vi "v5.3.vi"() -> ()   [LabVIEW 2018]
uses:
  <vilib>/DAQmx/read.llb/DAQmx Read (Analog 1D DBL NChan 1Samp).vi
  <extravilib>/ChannelInstances/Lossy Stream-c(a[.](c(dbl,dbl,dbl,dbl)),stamp,a[.](dbl),c(dbl,dbl,dbl,dbl,dbl,dbl,dbl))/Read With Abort.vi
  <extravilib>/ChannelInstances/High Speed Stream-c(a[.](c(dbl,dbl,dbl,dbl)),stamp,a[.](dbl),c(dbl,dbl,dbl,dbl,dbl,dbl,dbl))/_Read For Replicate.vi
  <extravilib>/ChannelInstances/Lossy Stream-c(a[.](c(dbl,dbl,dbl,dbl)),stamp,a[.](dbl),c(dbl,dbl,dbl,dbl,dbl,dbl,dbl))/Write With Abort.vi
  <extravilib>/ChannelInstances/Lossy Stream-c(a[.](c(dbl,dbl,dbl,dbl)),stamp,a[.](dbl),c(dbl,dbl,dbl,dbl,dbl,dbl,dbl))/EndpointRead.vi
  <extravilib>/ChannelInstances/Lossy Stream-c(a[.](c(dbl,dbl,dbl,dbl)),stamp,a[.](dbl),c(dbl,dbl,dbl,dbl,dbl,dbl,dbl))/Endpoint.vi
  <extravilib>/ChannelInstances/Lossy Stream-c(a[.](c(dbl,dbl,dbl,dbl)),stamp,a[.](dbl),c(dbl,dbl,dbl,dbl,dbl,dbl,dbl))/Instantiate.vi
  <extravilib>/ChannelInstances/Lossy Stream-c(a[.](c(dbl,dbl,dbl,dbl)),stamp,a[.](dbl),c(dbl,dbl,dbl,dbl,dbl,dbl,dbl))/)Channel.vi
  <resource>/ChannelSupport/_ChannelSupport/WaitIfNeeded.vi
  <extravilib>/ChannelInstances/High Speed Stream-c(a[.](c(dbl,dbl,dbl,dbl)),stamp,a[.](dbl),c(dbl,dbl,dbl,dbl,dbl,dbl,dbl))/Instantiate.vi
  <extravilib>/ChannelInstances/High Speed Stream-c(a[.](c(dbl,dbl,dbl,dbl)),stamp,a[.](dbl),c(dbl,dbl,dbl,dbl,dbl,dbl,dbl))/)Channel.vi
  <extravilib>/ChannelInstances/High Speed Stream-c(a[.](c(dbl,dbl,dbl,dbl)),stamp,a[.](dbl),c(dbl,dbl,dbl,dbl,dbl,dbl,dbl))/Abort Signal/Init Signal.vi
  <vilib>/Utility/file.llb/Write Delimited Spreadsheet (string).vi
  <vilib>/DAQmx/create/channels.llb/DAQmx Create Channel (AI-Temperature-Thermocouple).vi
  <vilib>/DAQmx/configure/timing.llb/DAQmx Timing (Sample Clock).vi
  <vilib>/DAQmx/miscellaneous.llb/DAQmx Fill In Error Info.vi
  <extravilib>/ChannelInstances/High Speed Stream-c(a[.](c(dbl,dbl,dbl,dbl)),stamp,a[.](dbl),c(dbl,dbl,dbl,dbl,dbl,dbl,dbl)).lvlib
  <resource>/objmgr/daqmx.rc
  <extravilib>/ChannelInstances/Lossy Stream-c(a[.](c(dbl,dbl,dbl,dbl)),stamp,a[.](dbl),c(dbl,dbl,dbl,dbl,dbl,dbl,dbl)).lvlib
panel:
  out "DAQ Current Time":timestamp format="%<%X>T"
  in  "UI Refresh Rate (Hz)":u32=1 min=1 max=500 step=1
  out "Line Pressures":T1(graph)
  in  "Boondoggle":dbl(slide) scale=0.0..10.0
  out "Line Temperatures":T1(graph)
  out "Stoichiometric AFR [g/s]":dbl
  in  "stop":bool
  in  "Species List":string[][](table)=[["Custom", "9999999999"], ["Methanol", "6.47"], ["Butanol", "11.2"], ["Diesel", "14.5"], ["Gasoline", "14.7"], ["Propane", "15.67"], ["Methane", "13.19"], ["Hydrogen", "34.3"], ["Ammonia", "6.0466"], ["Pentane", "15.32"], ["Butane", "14.98"], ["Hexane", "15.24"], ["Ethanol", "9"], ["Empty (Not Used)", "0"]]
  in  "Lines Tab Control\n(Don't delete)":enum32{"Live Data", "AFR Info", "Setup Lines"}(tab)
  out "Flowrate Data":T2(array[cluster])
  out "AFR Display":T3(array[cluster])
  in  "Line Setup":T4(array[cluster])
  out "Actual Sample Rate":dbl
  out "Export Timestamp":timestamp format="%<%H:%M:%S>T"
  out "Rig Temperatures":T5
  out "UI Timestamp":timestamp format="%<%X\n%x>T"
  in  "file path (dialog if empty)":path
  out "Export Loop Status":T6(ring)
  in  "Start Recording?":bool
  in  "Stop Recording?":bool
  out "Aquisition\nLoop Status":T7(ring)
  in  "OK Button":bool
  in  "DAQ Properties":cluster{"Sample Rate [Hz]":dbl}={"Sample Rate [Hz]"=1.0} {"Sample Rate [Hz]" min=1.0 max=500.0 step=1.0}
  # "Live \n Live Line Data"
  # "Air-to-Fuel Ratios for each Line"
  # "Line Setup"
  # "Rig Temperatures [ °C]"
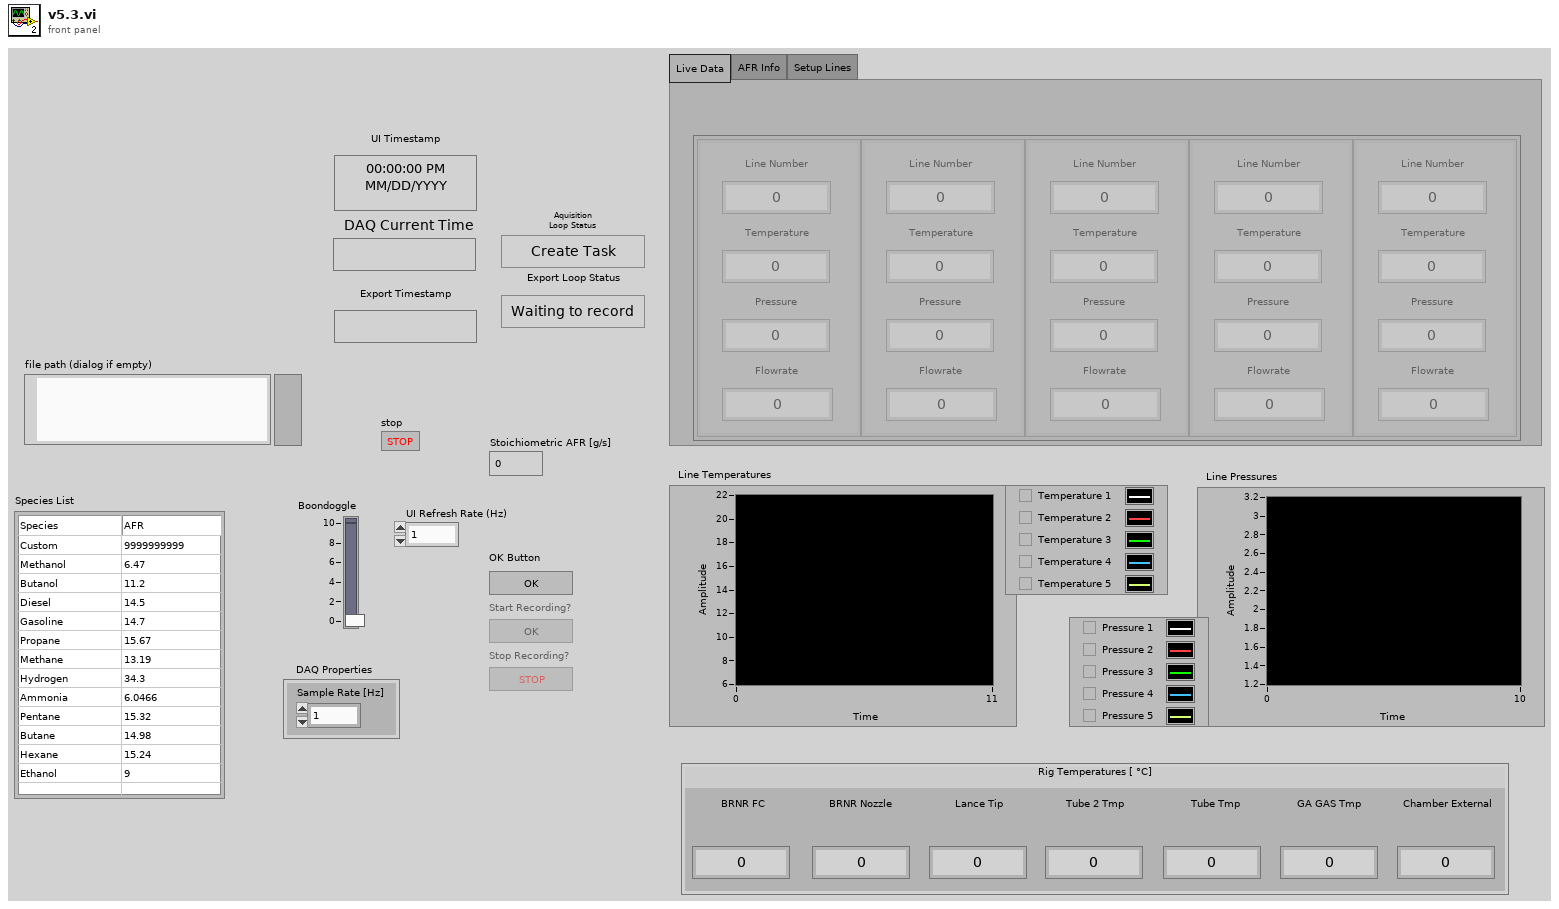
[diagram p1: front panel]
types:
  T1 = cluster{"[0]":dbl, "[1]":dbl, "[2]":dbl, "[3]":dbl, "[4]":dbl}
  T2 = cluster{"Line Number":dbl, "Temperature":dbl, "Pressure":dbl, "Flowrate":dbl}[]
  T3 = cluster{"Line Number":i32, "AFR":dbl, "Species":enum16{"Empty (Not used)", "Custom", "Methanol", "Ethanol", "Butanol", "Diesel", "Gasoline", "Propane", "Methane", "Hydrogen", "Pentane", "Butane", "Hexane"}}[]
  T4 = cluster{"Custom AFR":dbl, "Species":enum16{"Empty (Not used)", "Custom", "Methanol", "Ethanol", "Butanol", "Diesel", "Gasoline", "Propane", "Methane", "Hydrogen", "Pentane", "Butane", "Hexane"}}[]
  T5 = cluster{"BRNR FC":dbl, "BRNR Nozzle":dbl, "Lance Tip":dbl, "Tube 2 Tmp":dbl, "Tube Tmp":dbl, "GA GAS Tmp":dbl, "Chamber External":dbl}
  T6 = enum16{"Waiting to record", "Creating Spreadsheet", "Recording", "Finished Recording"}
  T7 = enum16{"Create Task", "Change Settings", "Check Settings", "Read Data", "End Task"}
  T8 = enum8{"Enabled", "Disabled", "Disabled and Grayed Out"}
  T9 = cluster{"Line":i32, "AFR":dbl, "Species":enum16{"Empty (Not used)", "Custom", "Methanol", "Ethanol", "Butanol", "Diesel", "Gasoline", "Propane", "Methane", "Hydrogen", "Pentane", "Butane", "Hexane"}}
  T10 = enum16{"Empty (Not used)", "Custom", "Methanol", "Ethanol", "Butanol", "Diesel", "Gasoline", "Propane", "Methane", "Hydrogen", "Pentane", "Butane", "Hexane"}
  T11 = cluster{"Flowrate Data":cluster{"Line Number":dbl, "Temperature":dbl, "Pressure":dbl, "Flowrate":dbl}[], "Current Time":timestamp, "DAQmx Data":dbl[], "Rig Temperatures":cluster{"BRNR FC":dbl, "BRNR Nozzle":dbl, "Lance Tip":dbl, "Tube 2 Tmp":dbl, "Tube Tmp":dbl, "GA GAS Tmp":dbl, "Chamber External Temp":dbl}}
  T12 = cluster{"BRNR FC":dbl, "BRNR Nozzle":dbl, "Lance Tip":dbl, "Tube 2 Tmp":dbl, "Tube Tmp":dbl, "GA GAS Tmp":dbl, "Chamber External Temp":dbl}
  T13 = typedef "High Speed Stream-c(a[.](c(dbl,dbl,dbl,dbl)),stamp,a[.](dbl),c(dbl,dbl,dbl,dbl,dbl,dbl,dbl)).lvlib/)Channel.ctl" = refnum<queue>
  T14 = typedef "Lossy Stream-c(a[.](c(dbl,dbl,dbl,dbl)),stamp,a[.](dbl),c(dbl,dbl,dbl,dbl,dbl,dbl,dbl)).lvlib/)Channel.ctl" = refnum<queue>
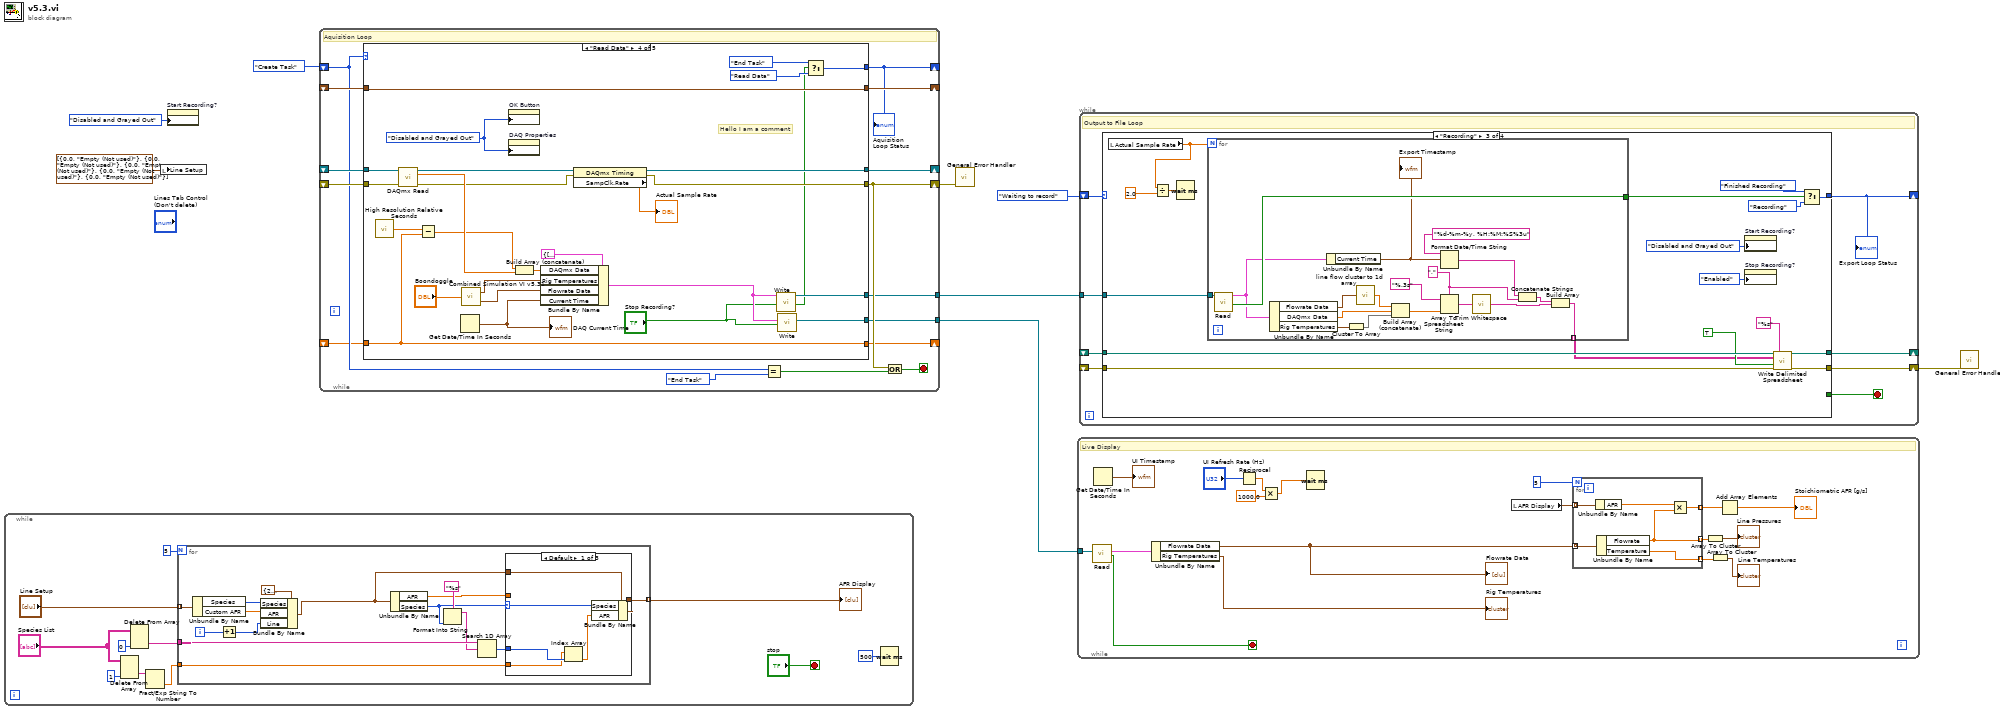
[diagram p0: block diagram]
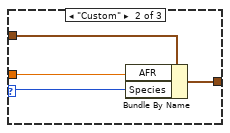
[diagram p2: hidden frame]
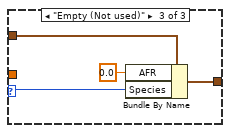
[diagram p3: hidden frame]
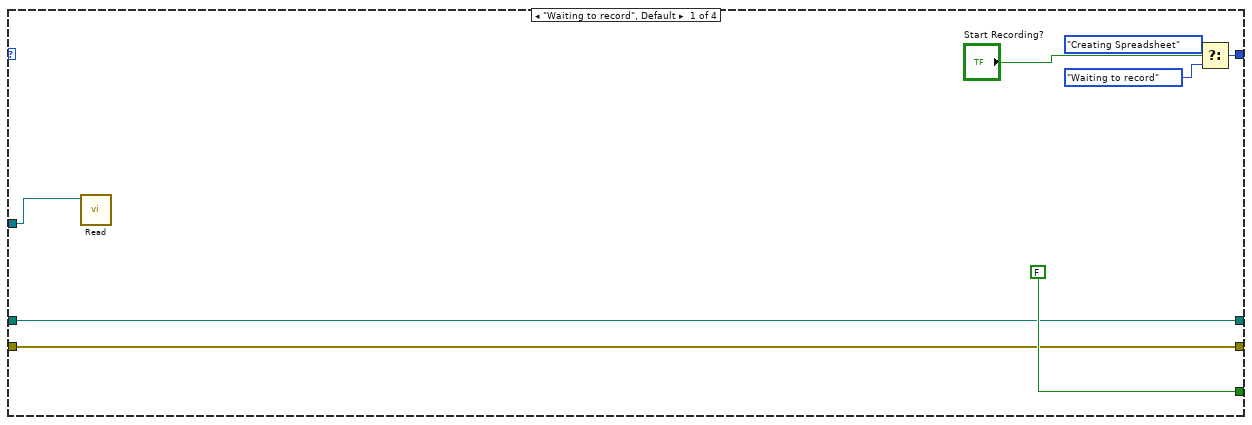
[diagram p4: hidden frame]
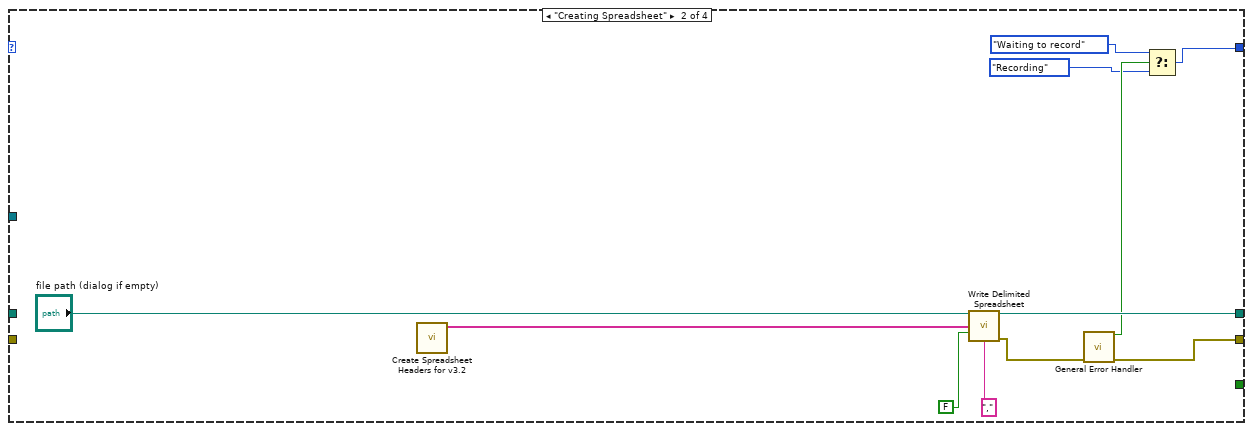
[diagram p5: hidden frame]
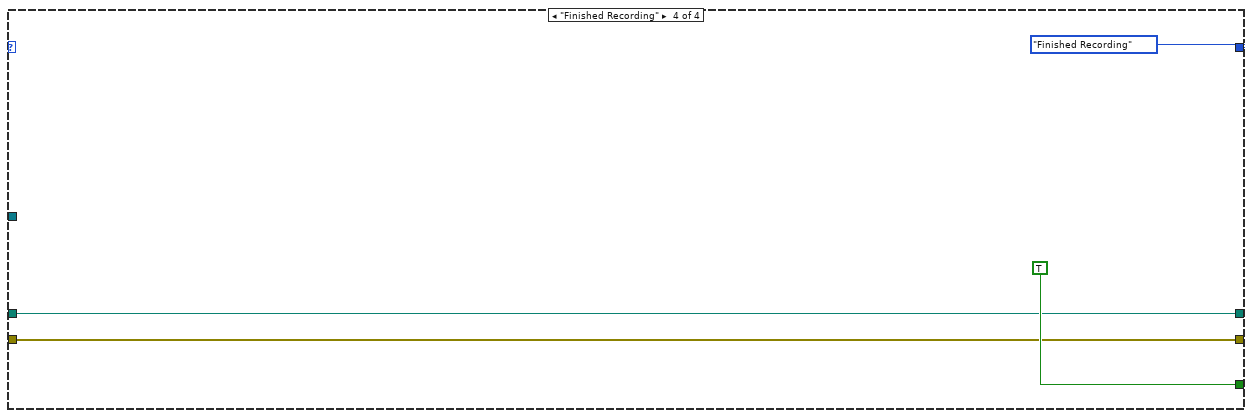
[diagram p6: hidden frame]
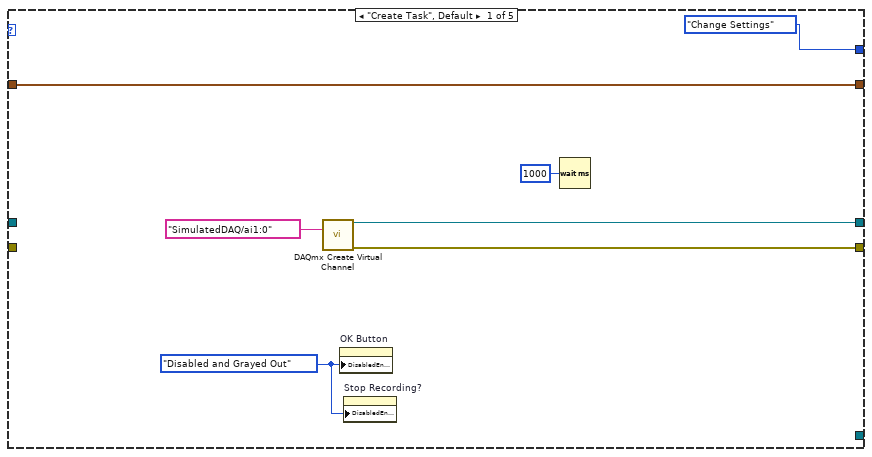
[diagram p7: hidden frame]
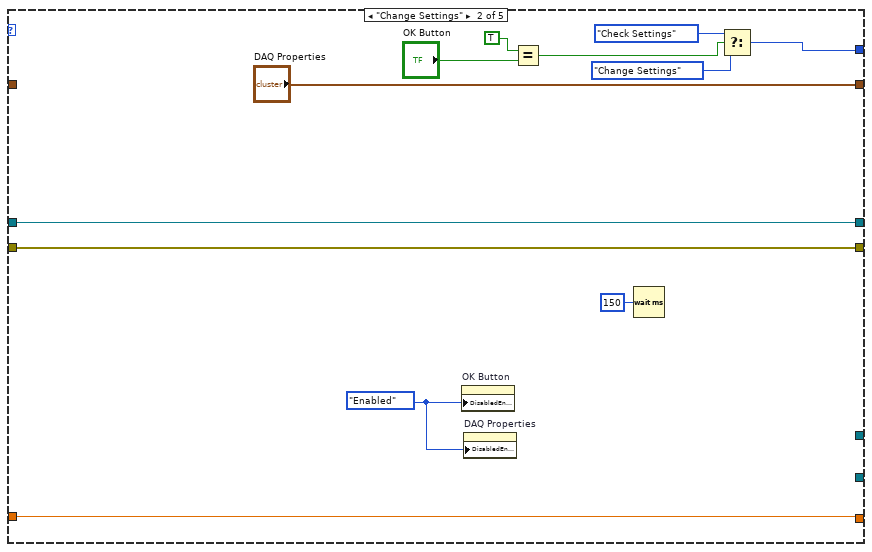
[diagram p8: hidden frame]
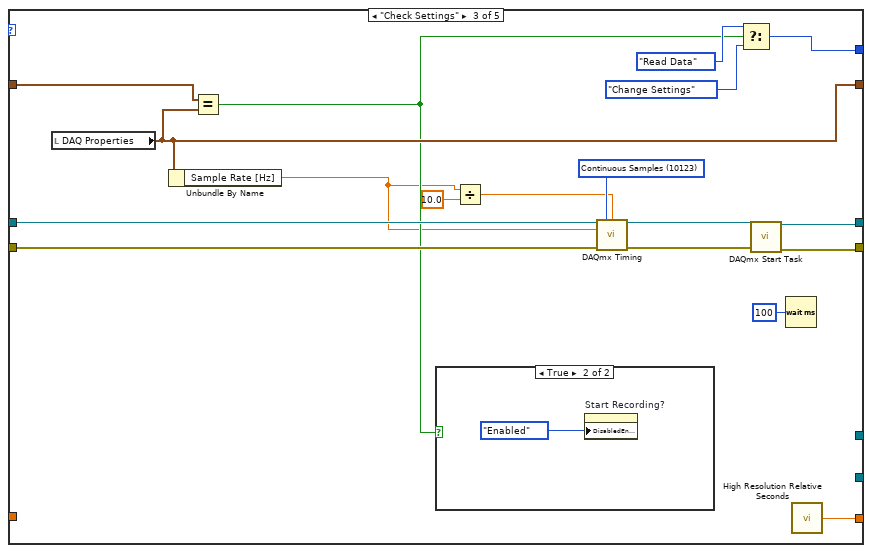
[diagram p9: hidden frame]
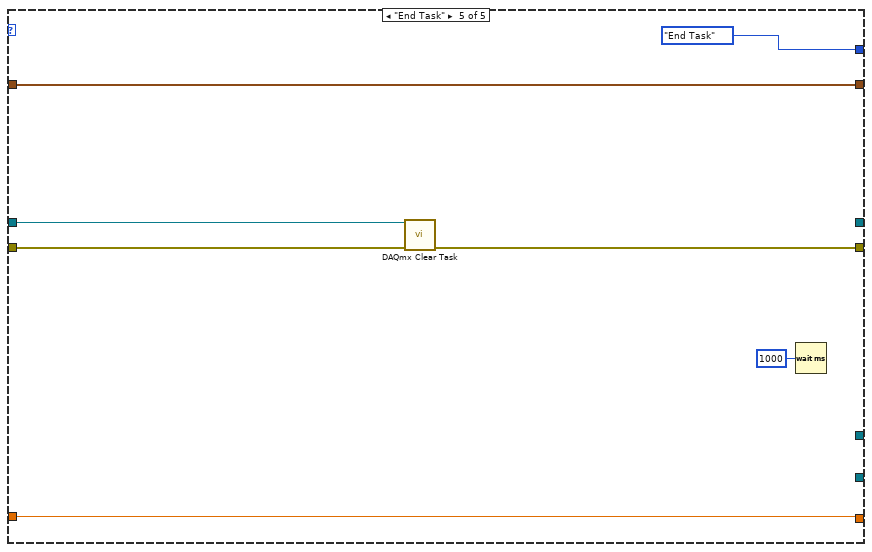
[diagram p11: hidden frame]
diagram:
  n1 = while {
    stop <- "stop" stop-if-true
    n2 = Delete From Array(array="Species List", index (col)=1 ("disabled index (col)")) -> (deleted portion=w14:string[])  [unwired: 2 in, 1 out]
    n3 = Delete From Array(array="Species List", index (col)=0) -> (deleted portion=w15:string[])  [unwired: 2 in, 1 out]
    n4 = Fract/Exp String To Number(string=w14) -> (number=w13:dbl[])  [unwired: 3 in, 1 out]
    n5 = for {
      N: 5 -> [_]
      tunnel: w15 -> [w33]
      tunnel: w13 -> [w30]
      tunnel: "Line Setup" -> [w23] mode=indexing
      tunnel: [w20] -> w9 mode=indexing
      i -> [w22]
      n6 = Unbundle By Name(w23) -> ("Species"=w27:T10, "Custom AFR"=w26:dbl)
      n7 = Increment(x=w22) -> (x+1=w24:i32)
      n8 = Bundle By Name(cluster=T9 {"Line"=2, "AFR"=1.0, "Species"=enum."Pentane"} ("AFR Inputs"), "Species"=w27, "AFR"=w26, "Line"=w24) -> (w21:T9)
      n9 = Unbundle By Name(w21) -> ("AFR"=w31:dbl, "Species"=w28:T10)
      n10 = Format Into String(format string="%s", w28) -> (resulting string=w32:string)  [unwired: 2 in, 1 out]
      n11 = Search 1D Array(1D array=w33, element=w32) -> (index of element=w29:i32)  [unwired: 1 in]
      n12 = case shown="Default" w28 {
        selector: w28 -> [w37 w41 w46]
        tunnel: w31 -> [_ w44 _]
        tunnel: w30 -> [w39 _ _]
        tunnel: w29 -> [w40 _ _]
        tunnel: [w35 w43 w48] -> w20
        tunnel: w21 -> [w36 w42 w47]
        frame Default {
          n13 = Index Array(array=w39, index=w40) -> (element=w38:dbl)
          n14 = Bundle By Name(cluster=w36, "Species"=w37, "AFR"=w38) -> (w35:T9)
        }
        frame "Custom" {
          n15 = Bundle By Name(cluster=w42, "AFR"=w44, "Species"=w41) -> (w43:T9)
        }
        frame "Empty (Not used)" {
          n16 = Bundle By Name(cluster=w47, "AFR"=0.0, "Species"=w46) -> (w48:T9)
        }
      }
    }
    "AFR Display" <- w9
    n17 = Wait (ms)(milliseconds to wait=u32 500) -> ()  [unwired: 1 out]
  }
  n18 = local write "Line Setup"(T4 [{"Custom AFR"=0.0, "Species"=enum."Empty (Not used)"}, {"Custom AFR"=0.0, "Species"=enum."Empty (Not used)"}, {"Custom AFR"=0.0, "Species"=enum."Empty (Not used)"}, {"Custom AFR"=0.0, "Species"=enum."Empty (Not used)"}, {"Custom AFR"=0.0, "Species"=enum."Empty (Not used)"}] ("Line Setup 2")) -> ()
  n19 = property on="Start Recording?" class="Bool"("DisabledEnum"=T8."Disabled and Grayed Out" ("Disabled")) -> ()  [unwired: 2 in, 2 out]
  n20 = while {
    shift-right: [w58] -> _
    shift-left: T7."Create Task" -> [w54]
    shift-right: [w63] -> _
    shift-left: _ -> [w61]
    shift-right: [w57] -> w4
    shift-left: _ -> [w60]
    shift-right: [w62] -> _
    shift-left: _ -> [w59]
    tunnel: [w53] -> w6
    tunnel: [w51] -> w2
    shift-right: [w49] -> _
    shift-left: _ -> [w50]
    stop <- w52 stop-if-true
    # "Aquisition Loop"
    n21 = case shown="\"Read Data\"" w54 {
      tunnel: [w70 w82 w90 w115 _] -> w63
      tunnel: [w69 w81 w89 w116 w135] -> w57
      tunnel: [T7."Change Settings" w75 w96 w124 T7."End Task"] -> w58
      tunnel: [w66 "DAQ Properties" w93 w126 w134] -> w62
      tunnel: w61 -> [_ w82 w95 w128 w132]
      tunnel: w60 -> [_ w81 w94 w127 w131]
      tunnel: w59 -> [w66 _ w100 w126 w134]
      tunnel: [_ _ _ w120 _] -> w53
      tunnel: [_ w71 w83 w111 w129] -> w49
      tunnel: w50 -> [_ w71 _ w111 w129]
      tunnel: [_ _ _ w108 _] -> w51
      frame "Create Task", Default {
        w64 = T8."Disabled and Grayed Out" ("Disabled")
        n22 = call-poly <vilib>:"DAQmx Create Virtual Channel.vi"("physical channels"=tag "SimulatedDAQ/ai1:0") -> ("task out"=w70:refnum<k21>, "error out"=w69:errorcluster)  [unwired: 13 in]
        n23 = property on="OK Button" class="Bool"("DisabledEnum"=w64) -> ()  [unwired: 2 in, 2 out]
        n24 = property on="Stop Recording?" class="Bool"("DisabledEnum"=w64) -> ()  [unwired: 2 in, 2 out]
        n25 = Wait (ms)(milliseconds to wait=u32 1000) -> ()  [unwired: 1 out]
      }
      frame "Change Settings" {
        w72 = T8."Enabled" ("Disabled")
        n26 = property on="OK Button" class="Bool"("DisabledEnum"=w72) -> ()  [unwired: 2 in, 2 out]
        n27 = property on="DAQ Properties" class="Clust (strict)"("DisabledEnum"=w72) -> ()  [unwired: 2 in, 2 out]
        n28 = Equal?(x=TRUE, y="OK Button") -> (x = y?=w77:bool)
        n29 = Wait (ms)(milliseconds to wait=u32 150) -> ()  [unwired: 1 out]
        n30 = Select(t=T7."Check Settings", s=w77, f=T7."Change Settings") -> (s? t:f=w75:T7)
      }
      frame "Check Settings" {
        w88 = 10123 items=["Finite Samples"=10178, "Continuous Samples"=10123, "Hardware Timed Single Point"=12522] ("sample mode")
        n31 = local read "DAQ Properties"() -> (w93:cluster{"Sample Rate [Hz]":dbl})
        n32 = Unbundle By Name(w93) -> ("Sample Rate [Hz]"=w85:dbl)
        n33 = Equal?(x=w100, y=w93) -> (x = y?=w87:bool)
        n34 = case shown="True" w87 {
          frame False {
          }
          frame True {
            n35 = property on="Start Recording?" class="Bool"("DisabledEnum"=T8."Enabled" ("Disabled")) -> ()  [unwired: 2 in, 2 out]
          }
        }
        n36 = Divide(x=w85, y=10.0) -> (x/y=w84:dbl)
        n37 = call-poly <vilib>:"DAQmx Timing.vi"("task/channels in"=w95, "sample mode"=w88, "samples per channel"=w84, "rate"=w85, "error in"=w94) -> ("task out"=w92:refnum<k21>, "error out"=w91:errorcluster)  [unwired: 9 in]
        n38 = Select(t=T7."Read Data", s=w87, f=T7."Change Settings") -> (s? t:f=w96:T7)
        n39 = call <vilib>:"DAQmx Start Task.vi"("task/channels in"=w92, "error in"=w91) -> ("task out"=w90:refnum<k21>, "error out"=w89:errorcluster)  [unwired: 12 in]
        n40 = Wait (ms)(milliseconds to wait=u32 100) -> ()  [unwired: 1 out]
        n41 = call <vilib>:"High Resolution Relative Seconds.vi"() -> ("relative seconds"=w83:dbl)
      }
      frame "Read Data" {
        w119 = T8."Disabled and Grayed Out" ("Disabled")
        # "Hello I am a comment"
        n42 = call <vilib>:"High Resolution Relative Seconds.vi"() -> ("relative seconds"=w113:dbl)
        n43 = call-poly <vilib>:"DAQmx Read.vi"("task/channels in"=w128, "error in"=w127) -> ("task out"=w117:refnum<k21>, "data"=w122:dbl[], "error out"=w114:errorcluster)  [unwired: 11 in]
        n44 = Subtract(x=w113, y=w111) -> (x-y=w112:dbl)
        n45 = Get Date/Time In Seconds() -> (seconds since 1Jan1904=w103:timestamp)
        "DAQ Current Time" <- w103
        n46 = call "Combined Simulation VI v5.31.vi"("Boondoggle Input"="Boondoggle") -> ("Rig Temperatures Cluster"=w102:T12, "Line Data (Array of Clusters)"=w104:T2)
        n47 = property on="OK Button" class="Bool"("DisabledEnum"=w119) -> ()  [unwired: 2 in, 2 out]
        n48 = property on="DAQ Properties" class="Clust (strict)"("DisabledEnum"=w119) -> ()  [unwired: 2 in, 2 out]
        n49 = Build Array (concatenate)(w112, w122) -> (w106:dbl[])
        n50 = Bundle By Name(cluster=T11 {"Flowrate Data"=[{"Line Number"=1.0, "Temperature"=17.480721541683437, "Pressure"=24.0, "Flowrate"=0.0}, {"Line Number"=2.0, "Temperature"=21.850901927104296, "Pressure"=30.0, "Flowrate"=0.0}, {"Line Number"=3.0, "Temperature"=26.221082312525155, "Pressure"=36.0, "Flowrate"=0.0}, {"Line Number"=4.0, "Temperature"=30.591262697946018, "Pressure"=42.00000000000001, "Flowrate"=0.0}, {"Line Number"=5.0, "Temperature"=34.96144308336687, "Pressure"=48.0, "Flowrate"=0.0}], "Current Time"=timestamp(0 s since 1904-01-01), "DAQmx Data"=[], "Rig Temperatures"={"BRNR FC"=0.0, "BRNR Nozzle"=0.0, "Lance Tip"=0.0, "Tube 2 Tmp"=0.0, "Tube Tmp"=0.0, "GA GAS Tmp"=0.0, "Chamber External Temp"=0.0}}, "DAQmx Data"=w106, "Rig Temperatures"=w102, "Flowrate Data"=w104, "Current Time"=w103) -> (w118:T11)
        n51 = property class="DAQmx Timing"(reference=w117, error in=w114) -> (reference out=w115:refnum<k21>, error out=w116:errorcluster, "SampClk.Rate"=→"Actual Sample Rate":dbl)
        n52 = call <extravilib>:"Write.vi"("last element? (F)"="Stop Recording?", "element"=w118) -> ("done?"=w107:bool, "channel"=w120:T13)  [unwired: 7 in, 1 out]
        n53 = call <extravilib>:"Write.vi"("last element? (F)"="Stop Recording?", "element"=w118) -> ("channel"=w108:T14)  [unwired: 7 in, 2 out]
        n54 = Select(t=T7."End Task", s=w107, f=T7."Read Data") -> (s? t:f=w124:T7)
      }
      frame "End Task" {
        n55 = call <vilib>:"DAQmx Clear Task.vi"("task in"=w132, "error in"=w131) -> ("error out"=w135:errorcluster)  [unwired: 13 in]
        n56 = Wait (ms)(milliseconds to wait=u32 1000) -> ()  [unwired: 1 out]
      }
    }
    "Aquisition\nLoop Status" <- w58
    n57 = Equal?(x=w54, y=T7."End Task") -> (x = y?=w55:bool)
    n58 = Or(x=w57, y=w55) -> (x .or. y?=w52:bool)
  }
  n59 = call <vilib>:"General Error Handler.vi"("error in (no error)"=w4) -> ()  [unwired: 10 in, 5 out]
  n60 = while {
    tunnel: w2 -> [w144]
    stop <- w140 stop-if-true
    # "Live Display"
    n61 = call <extravilib>:"Read.vi"("channel"=w144) -> ("last element?"=w140:bool, "element"=w143:T11)  [unwired: 5 in, 4 out]
    n62 = Get Date/Time In Seconds() -> (seconds since 1Jan1904=→"UI Timestamp":timestamp)
    n63 = Unbundle By Name(w143) -> ("Flowrate Data"=w141:T2, "Rig Temperatures"=→"Rig Temperatures":T12)
    "Flowrate Data" <- w141
    n64 = Reciprocal(x="UI Refresh Rate (Hz)") -> (1/x=w137:dbl)
    n65 = Multiply(x=w137, y=1000.0) -> (x*y=w136:dbl)
    n66 = Wait (ms)(milliseconds to wait=w136) -> ()  [unwired: 1 out]
    n67 = local read "AFR Display"() -> (w151:T3)
    n68 = for {
      N: 5 -> [_]
      tunnel: w151 -> [w159] mode=indexing
      tunnel: [w157] -> w150 mode=indexing
      tunnel: [w156] -> w147 mode=indexing
      tunnel: [w155] -> w148 mode=indexing
      tunnel: w141 -> [w154] mode=indexing
      n69 = Unbundle By Name(w159) -> ("AFR"=w158:dbl)
      n70 = Unbundle By Name(w154) -> ("Flowrate"=w155:dbl, "Temperature"=w156:dbl)
      n71 = Multiply(x=w158, y=w155) -> (x*y=w157:dbl)
    }
    n72 = Array To Cluster(array=w148) -> (cluster=→"Line Pressures":T1)
    n73 = Array To Cluster(array=w147) -> (cluster=→"Line Temperatures":T1)
    n74 = Add Array Elements(numeric array=w150) -> (sum=→"Stoichiometric AFR [g/s]":dbl)
  }
  n75 = while {
    shift-right: [w167] -> _
    shift-left: T6."Waiting to record" -> [w166]
    tunnel: w6 -> [w164]
    shift-right: [w162] -> _
    shift-left: _ -> [w163]
    shift-right: [w161] -> w5
    shift-left: _ -> [w160]
    stop <- w165 stop-if-true
    # "Output to File Loop"
    n76 = case shown="\"Recording\"" w166 {
      tunnel: [w172 w178 w202 T6."Finished Recording"] -> w167
      tunnel: [FALSE _ _ TRUE] -> w165
      tunnel: w164 -> [w168 _ w199 _]
      tunnel: w163 -> [w170 _ w196 w223]
      tunnel: [w170 w186 w197 w223] -> w162
      tunnel: [w169 w180 w192 w222] -> w161
      tunnel: w160 -> [w169 _ w195 w222]
      frame "Waiting to record", Default {
        n77 = call <extravilib>:"Read.vi"("channel"=w168) -> ()  [unwired: 6 in, 5 out]
        n78 = Select(t=T6."Creating Spreadsheet", s="Start Recording?", f=T6."Waiting to record") -> (s? t:f=w172:T6)
      }
      frame "Creating Spreadsheet" {
        n79 = call "Create Spreadsheet Headers for v3.2.vi"() -> ("Array"=w185:string[])  [unwired: 11 in]
        n80 = call-poly <vilib>:"Write Delimited Spreadsheet.vi"("file path (dialog if empty)"="file path (dialog if empty)", "1D data"=w185, "append to file? (new file:F)"=FALSE, "delimiter (\\t)"="," ("delimiter (\\t)")) -> ("new file path (Not A Path if cancelled)"=w186:path, "error out"=w181:errorcluster)  [unwired: 10 in]
        n81 = call <vilib>:"General Error Handler.vi"("error in (no error)"=w181) -> ("error?"=w179:bool, "error out"=w180:errorcluster)  [unwired: 10 in, 3 out]
        n82 = Select(t=T6."Waiting to record", s=w179, f=T6."Recording") -> (s? t:f=w178:T6)
      }
      frame "Recording" {
        n83 = local read "Actual Sample Rate"() -> (w188:dbl)
        n84 = Divide(x=w188, y=2.0) -> (x/y=w187:dbl)
        n85 = Wait (ms)(milliseconds to wait=w187) -> ()  [unwired: 1 out]
        n86 = for {
          N: w188 -> [_]
          tunnel: w199 -> [w220]
          tunnel: [w219] -> w198
          tunnel: [w204] -> w190 mode=indexing
          w209 = "," ("delimiter (Tab)")
          n87 = call <extravilib>:"Read.vi"("channel"=w220) -> ("done?"=w219:bool, "element"=w217:T11)  [unwired: 6 in, 3 out]
          n88 = Unbundle By Name(w217) -> ("Flowrate Data"=w218:T2, "DAQmx Data"=w215:dbl[], "Rig Temperatures"=w221:T12)
          n89 = Unbundle By Name(w217) -> ("Current Time"=w210:timestamp)
          "Export Timestamp" <- w210
          n90 = Cluster To Array(cluster=w221) -> (array=w216:dbl[])
          n91 = call "line flow cluster to 1d array.vi"("Flowrate Data"=w218) -> ("Array"=w214:dbl[])
          n92 = Build Array (concatenate)(w214, w215, w216) -> (w207:dbl[])
          n93 = Format Date/Time String(time format string (%c)="%d-%m-%y, %H:%M:%S%3u", seconds (now)=w210) -> (date/time string=w208:string)  [unwired: 1 in]
          n94 = Array To Spreadsheet String(delimiter (Tab)=w209, array=w207, 3:"%.3s" ("format string")) -> (spreadsheet string=w213:string)
          n95 = call <vilib>:"Trim Whitespace.vi"("string"=w213) -> ("trimmed string"=w205:string)  [unwired: 1 in]
          n96 = Concatenate Strings(w208, w209) -> (w206:string)
          n97 = Build Array(w206, w205) -> (w204:string[])
        }
        n98 = property on="Start Recording?" class="Bool"("DisabledEnum"=T8."Disabled and Grayed Out" ("Disabled")) -> ()  [unwired: 2 in, 2 out]
        n99 = property on="Stop Recording?" class="Bool"("DisabledEnum"=T8."Enabled" ("Disabled")) -> ()  [unwired: 2 in, 2 out]
        n100 = call-poly <vilib>:"Write Delimited Spreadsheet.vi"("file path (dialog if empty)"=w196, "format (%s)"="%s", "2D data"=w190, "append to file? (new file:F)"=TRUE, "error in (no error)"=w195) -> ("new file path (Not A Path if cancelled)"=w197:path, "error out"=w192:errorcluster)  [unwired: 9 in]
        n101 = Select(t=T6."Finished Recording", s=w198, f=T6."Recording") -> (s? t:f=w202:T6)
      }
      frame "Finished Recording" {
      }
    }
    "Export Loop Status" <- w167
  }
  n102 = call <vilib>:"General Error Handler.vi"("error in (no error)"=w5) -> ()  [unwired: 10 in, 5 out]
